vi "SubVI.vi"() -> ()   [LabVIEW 2023]
panel:
  in  "Fahrenheit":dbl
  out "Centigrade":dbl
  in  "stop":bool
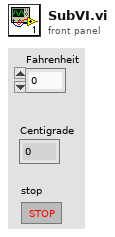
[diagram p1: front panel]
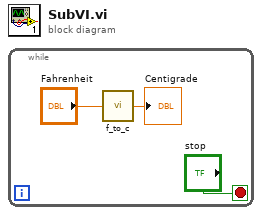
[diagram p0: block diagram]
diagram:
  n1 = while {
    stop <- "stop" stop-if-true
    n2 = call "f_to_c.vi"("Fahrenheit Temperature"="Fahrenheit") -> ("Celsius Temperature"=→"Centigrade":dbl)
  }
